vi "ConvertWorldProperties.vi"(5 "Reply":string) -> (1 "Poses":T2(array[cluster]) {"Point"."y" format="%#_3f"}, 2 "Twists":T1(array[cluster]), 3 "error out":errorcluster, 4 "names":string[](array[string]))   [LabVIEW 2010]
uses:
  ROS/parsing/std_msgs/subs/parse_string_array.vi
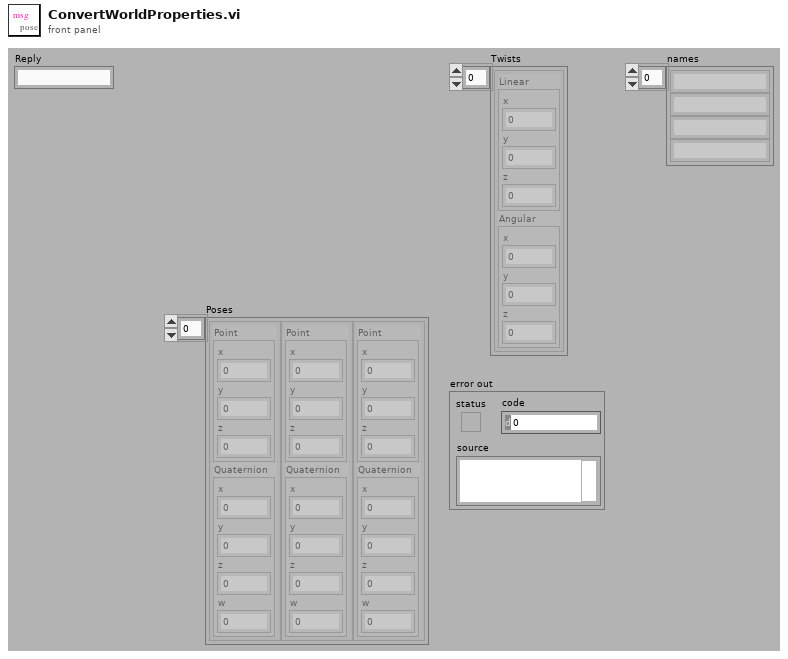
[diagram p1: front panel]
types:
  T1 = cluster{"Linear":cluster{"x":dbl, "y":dbl, "z":dbl}, "Angular":cluster{"x":dbl, "y":dbl, "z":dbl}}[]
  T2 = cluster{"Point":cluster{"x":dbl, "y":dbl, "z":dbl}, "Quaternion":cluster{"x":dbl, "y":dbl, "z":dbl, "w":dbl}}[]
  T3 = cluster{"Point":cluster{"x":dbl, "y":dbl, "z":dbl}, "Quaternion":cluster{"x":dbl, "y":dbl, "z":dbl, "w":dbl}}
  T4 = cluster{"Linear":cluster{"x":dbl, "y":dbl, "z":dbl}, "Angular":cluster{"x":dbl, "y":dbl, "z":dbl}}
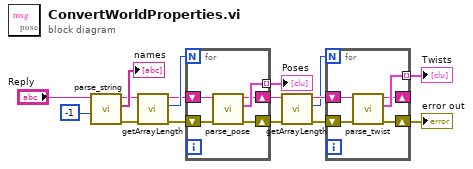
[diagram p0: block diagram]
diagram:
  n1 = call-poly "parse_string.vi"("Array Size"=-1, "msg in"="Reply") -> ("error out"=w12:errorcluster, "strings"=→"names":string[], "msg out"=w1:string)  [unwired: 3 in]
  n2 = call "getArrayLength.vi"("error in"=w12, "msg in"=w1) -> ("error out"=w13:errorcluster, "array length"=w3:u32, "msg out"=w2:string)  [unwired: 3 in]
  n3 = for {
    N: w3 -> [_]
    tunnel: [w20] -> w7 mode=indexing
    shift-right: [w19] -> w6
    shift-left: w2 -> [w21]
    shift-right: [w17] -> w14
    shift-left: w13 -> [w18]
    n4 = call "parse_pose.vi"("error in"=w18, "msg in"=w21) -> ("error out"=w17:errorcluster, "Pose"=w20:T3, "msg out"=w19:string)  [unwired: 3 in]
  }
  "Poses" <- w7
  n5 = call "getArrayLength.vi"("error in"=w14, "msg in"=w6) -> ("error out"=w15:errorcluster, "array length"=w4:u32, "msg out"=w5:string)  [unwired: 3 in]
  n6 = for {
    N: w4 -> [_]
    tunnel: [w25] -> w8 mode=indexing
    shift-right: [w24] -> _
    shift-left: w5 -> [w26]
    shift-right: [w22] -> w16
    shift-left: w15 -> [w23]
    n7 = call "parse_twist.vi"("error in"=w23, "msg in"=w26) -> ("error out"=w22:errorcluster, "Twist"=w25:T4, "msg out"=w24:string)  [unwired: 3 in]
  }
  "error out" <- w16
  "Twists" <- w8
